vi "Peroid Read.vi"(4 "error in (no error)":errorcluster, 6 "Container State":T4, 7 "Display State In":T1) -> (0 "error out":errorcluster, 2 "Value":cluster{"start":timestamp, "end":timestamp} {"start" format="%<%H:%M:%S\n%x>T"; "end" format="%<%H:%M:%S\n%x>T"}, 3 "Display State Out":T1)   [LabVIEW 2013, in "UI_TimeSelector.xctl"]
uses:
  UI_TimeSelector.xctl
  <vilib>/_xctls/Container State.ctl
  State.ctl
  Typedefs/INTERNAL-DATA.ctl
  Interface/DEF-Mode.ctl
  <vilib>/_xctls/XControlSupport.lvlib
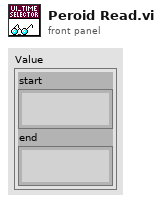
[diagram p1: front panel]
types:
  T1 = typedef "UI_TimeSelector.xctl/State.ctl" = cluster{"data":T2, "mode":T3}
  T2 = typedef "UI_TimeSelector.xctl/INTERNAL-DATA.ctl" = cluster{"year":string, "month":string, "day":string, "hour":string, "minute":string, "second":string}
  T3 = typedef "UI_TimeSelector.xctl/DEF-Mode.ctl" = enum16{"YYYYMMDDHHMM", "YYYYMMDDHHMMSS", "YYYY", "YYYYMM", "YYYYMMDD", "HHMM", "HHMMSS"}
  T4 = typedef "XControlSupport.lvlib/Container State.ctl" = cluster{"Indicator?":bool, "Run Mode?":bool, " Refnum":refnum<vi>}
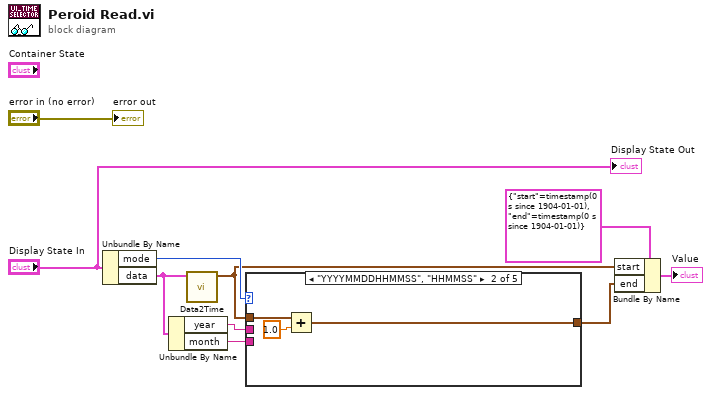
[diagram p0: block diagram]
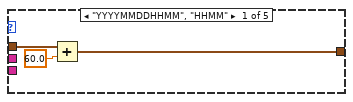
[diagram p2: hidden frame]
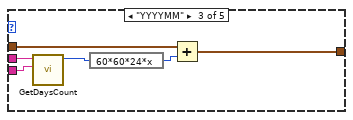
[diagram p3: hidden frame]
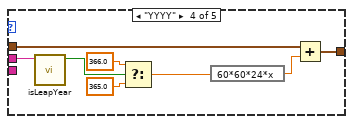
[diagram p4: hidden frame]
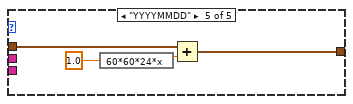
[diagram p5: hidden frame]
diagram:
  n1 = Unbundle By Name("Display State In") -> ("mode"=w8:T3, "data"=w3:T2)
  n2 = Unbundle By Name(w3) -> ("year"=w2:string, "month"=w1:string)
  n3 = call "Data2Time.vi"("data"=w3) -> ("Time"=w6:timestamp)  [unwired: 10 in]
  n4 = case shown="\"YYYYMMDDHHMMSS\", \"HHMMSS\"" w8 {
    tunnel: w6 -> [w12 w16 w22 w29 w34]
    tunnel: [w11 w14 w19 w24 w32] -> w4
    tunnel: w2 -> [_ _ w18 w23 _]
    tunnel: w1 -> [_ _ w17 _ _]
    frame "YYYYMMDDHHMM", "HHMM" {
      n5 = Add(x=w12, y=60.0) -> (x+y=w11:timestamp)
    }
    frame "YYYYMMDDHHMMSS", "HHMMSS" {
      n6 = Add(x=w16, y=1.0) -> (x+y=w14:timestamp)
    }
    frame "YYYYMM" {
      n7 = call "GetDaysCount.vi"("month"=w17, "year"=w18) -> ("Numeric"=w21:i32)  [unwired: 9 in]
      n8 = expression code="60*60*24*x"(w21) -> (w20:i32)
      n9 = Add(x=w22, y=w20) -> (x+y=w19:timestamp)
    }
    frame "YYYY" {
      n10 = call "isLeapYear.vi"("year"=w23) -> ("Boolean"=w28:bool)  [unwired: 10 in]
      n11 = Select(t=366.0, s=w28, f=365.0 ("t")) -> (s? t:f=w27:dbl)
      n12 = expression code="60*60*24*x"(w27) -> (w30:dbl)
      n13 = Add(x=w29, y=w30) -> (x+y=w24:timestamp)
    }
    frame "YYYYMMDD" {
      n14 = expression code="60*60*24*x"(1.0) -> (w33:dbl)
      n15 = Add(x=w34, y=w33) -> (x+y=w32:timestamp)
    }
  }
  n16 = Bundle By Name(cluster=cluster{"start":timestamp, "end":timestamp} {"start"=timestamp(0 s since 1904-01-01), "end"=timestamp(0 s since 1904-01-01)} ("Value"), "start"=w6, "end"=w4) -> (→"Value":cluster{"start":timestamp, "end":timestamp})
  "error out" <- "error in (no error)"
  "Display State Out" <- "Display State In"
